vi "Main.vi"() -> ()   [LabVIEW 2019]
panel:
  in  "Error In":errorcluster
  out "error_out":errorcluster
  out "tb_read_datetime":string
  out "tb_read":string
  in  "tf_exit":bool
  out "tf_status":bool
  in  "visa_device":refnum<visa-resource-name>
  # "Serial Read from a subvi using control references"
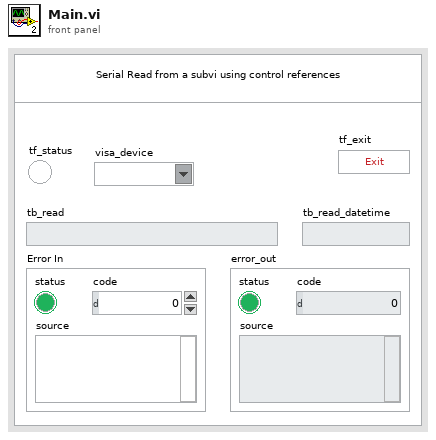
[diagram p1: front panel]
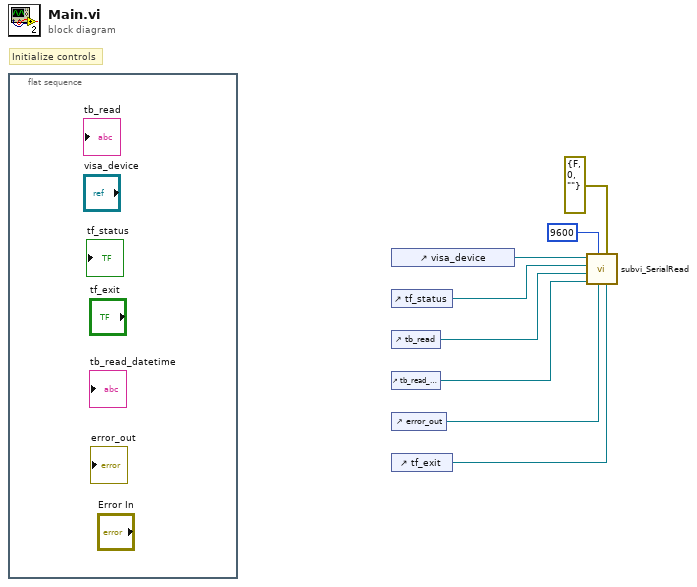
[diagram p0: block diagram]
diagram:
  # "Initialize controls"
  n1 = flat-sequence {
    frame #0 {
    }
  }
  n2 = control-ref of="visa_device"() -> (w6:refnum<vi>)
  n3 = control-ref of="tf_status"() -> (w5:refnum<vi>)
  n4 = control-ref of="tb_read"() -> (w4:refnum<vi>)
  n5 = control-ref of="tb_read_datetime"() -> (w3:refnum<vi>)
  n6 = control-ref of="error_out"() -> (w2:refnum<vi>)
  n7 = control-ref of="tf_exit"() -> (w1:refnum<vi>)
  n8 = call "subvi_SerialRead.vi"("tf_exit(Refnum)"=w1, "Error In"=errorcluster {"status"=FALSE, "code"=0, "source"=""}, "error_out(Refnum)"=w2, "baud_rate"=u32 9600, "tb_read_datetime(Refnum)"=w3, "tb_read(Refnum)"=w4, "tf_status(Refnum)"=w5, "visa_device(Refnum)"=w6) -> ()  [unwired: 4 in]
